vi "HouseBlend_Create.vi"(0 "reference in":refnum<class "HouseBlend.lvclass">, 5 "error in (no error)":errorcluster) -> (14 "reference out":refnum<class "HouseBlend.lvclass">, 19 "error out":errorcluster)   [LabVIEW 2020, in "HouseBlend.lvclass"]
uses:
  HouseBlend.lvclass
  C:/Projects/DesignPatterns/DecoratorPattern/Beverage_class/Beverage.lvclass
  Beverage_class/Beverage.lvclass
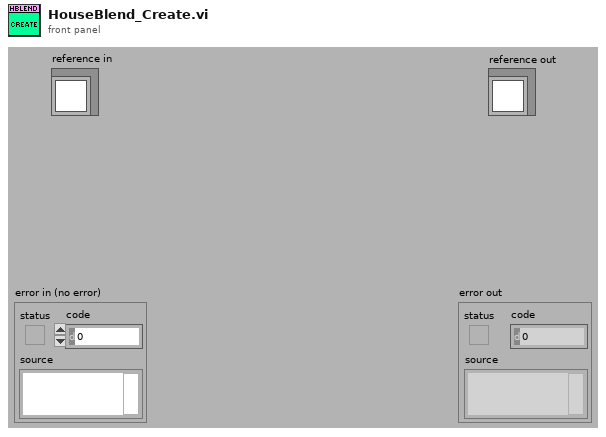
[diagram p1: front panel]
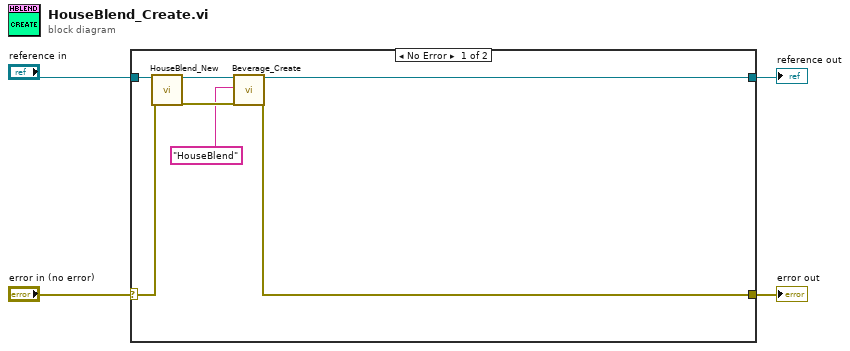
[diagram p0: block diagram]
diagram:
  n1 = case shown="No Error" "error in (no error)" {
    selector: "error in (no error)" -> [w10 w13]
    tunnel: [w5 w13] -> w3
    tunnel: "reference in" -> [w11 w12]
    tunnel: [w7 w12] -> w1
    frame No Error {
      n2 = call "HouseBlend_New.vi"("reference in"=w11, "error in (no error)"=w10) -> ("reference out"=w9:refnum<class "HouseBlend.lvclass">, "error out"=w8:errorcluster)  [unwired: 14 in, 2 out]
      n3 = call "Beverage_Create.vi"("reference in"=w9, "Description"="HouseBlend", "error in (no error)"=w8) -> ("reference out"=w7:refnum<class "HouseBlend.lvclass">, "error out"=w5:errorcluster)  [unwired: 15 in]
    }
    frame Error {
    }
  }
  "error out" <- w3
  "reference out" <- w1
